vi "Stage_int.vi"() -> ()   [LabVIEW 2015]
panel:
  in  "Group Name":string
  in  "IP Address":string
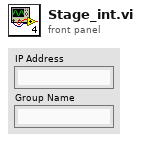
[diagram p1: front panel]
types:
  T1 = cluster{"connection TCP":refnum<k5>, "LogTo File":bool, "Log File refnum":refnum<file>, "no error if error log":bool}
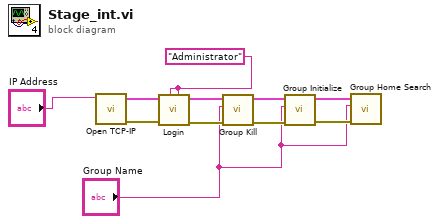
[diagram p0: block diagram]
diagram:
  w2 = "Administrator"
  n1 = call <userlib>:"Open TCP-IP.vi"("IP address"="IP Address") -> ("error out"=w6:errorcluster, "Connection ID"=w10:T1)  [unwired: 8 in, 1 out]
  n2 = call <userlib>:"Login.vi"("Password"=w2, "User"=w2, "error in (no error)"=w6, "connection ID in"=w10) -> ("error out"=w5:errorcluster, "connection ID out"=w9:T1)  [unwired: 5 in, 1 out]
  n3 = call <userlib>:"Group Kill.vi"("error in (no error)"=w5, "Group Name (250 c max)"="Group Name", "connection ID in"=w9) -> ("error out"=w4:errorcluster, "connection ID out"=w8:T1)  [unwired: 6 in, 1 out]
  n4 = call <userlib>:"Group Initialize.vi"("error in (no error)"=w4, "Group Name (250 c max)"="Group Name", "connection ID in"=w8) -> ("error out"=w3:errorcluster, "connection ID out"=w7:T1)  [unwired: 6 in, 1 out]
  n5 = call <userlib>:"Group Home Search.vi"("error in (no error)"=w3, "Group Name (250 c max)"="Group Name", "connection ID in"=w7) -> ()  [unwired: 6 in, 3 out]
